vi "register.private_lua.vi"(5 "LuaVIEW reference":T1) -> (15 "error out":errorcluster)   [LabVIEW 2012]
doc: "Registers a LuaVIEW function VI with the private registry of the current script's LuaVIEW state. When this function returns, the function is callable by scripts executing on the state's VM instance. When a VI with the same name is already in memory that VI will be registered, otherwise an attempt will be made to load the function VI from disk. If the path is relative, the function VI is assumed to be located relative to the resource base path. If the application is built and the function VI could not be located at the specified path, the VIs built into the application executable will be searched. The function is unregistered, and its VI reference closed, when the LuaVIEW state of the script is closed. The function VI will unload when no further references to it remain open. Note that the function manager displays a use count for privately registered functions.\nParameters:\nstr:path, path to the function VI.\nErrors:\nFunction name invalid.\nCould not load function VI.\nFunction VI has an invalid connector pane.\nFunction improperly documented."
uses:
  typedefs/t_LuaVIEW Reference.ctl
  subvis/private/LuaVIEW Pull (path).vi
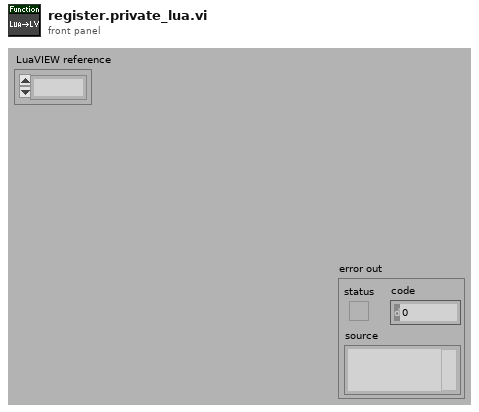
[diagram p1: front panel]
types:
  T1 = typedef "t_LuaVIEW Reference.ctl" = refnum<k1>
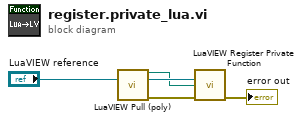
[diagram p0: block diagram]
diagram:
  n1 = call-poly "LuaVIEW Pull (poly).vi"("LuaVIEW reference in"="LuaVIEW reference") -> ("path"=w1:path, "LuaVIEW reference out"=w2:T1, "error out"=w3:errorcluster)  [unwired: 12 in]
  n2 = call "LuaVIEW Register Private Function.vi"("LuaVIEW reference in"=w2, "function VI path"=w1, "error in (no error)"=w3) -> ("error out"=→"error out":errorcluster)  [unwired: 11 in, 1 out]
